vi "doubleshutter_imagesplit.vi"(0 "image array":dbl[][](array[numeric]), 1 "DoubleShutter?":bool, 3 "x bin":dbl) -> (5 "lower half - atoms":dbl[][](graph), 6 "upper half - background":dbl[][](graph), 7 "Uncut Image":dbl[][](graph))   [LabVIEW 2013]
panel:
  in  "y bin":dbl
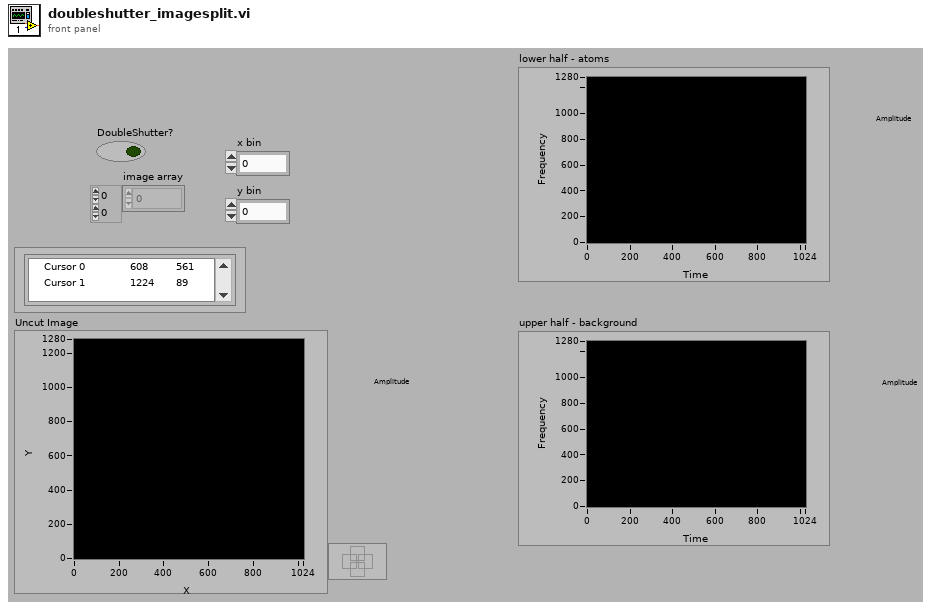
[diagram p1: front panel]
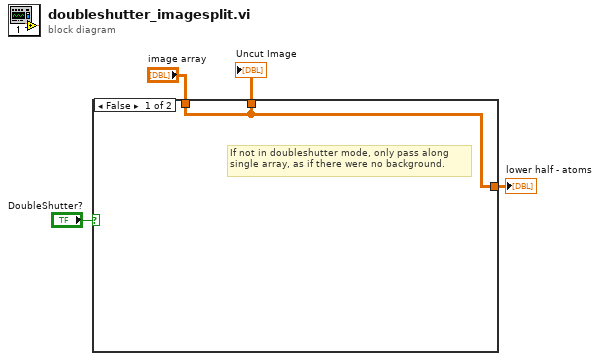
[diagram p0: block diagram]
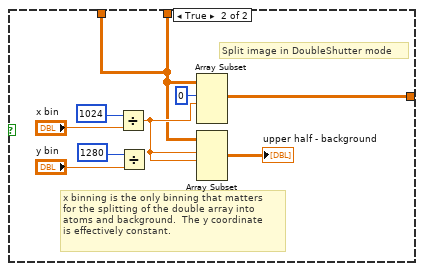
[diagram p2: hidden frame]
diagram:
  n1 = case shown="False" "DoubleShutter?" {
    tunnel: [w5 w8] -> w4
    tunnel: "image array" -> [w5 w8]
    tunnel: [w5 w7] -> w1
    frame False {
      # "If not in doubleshutter mode, only pass along\nsingle array, as if there were no background."
    }
    frame True {
      # "Split image in DoubleShutter mode"
      # "x binning is the only binning that matters\nfor the splitting of the double array into\natoms and background.  The y coordinate\nis effectively constant."
      n2 = Divide(x=1024 ("length"), y="x bin") -> (x/y=w12:dbl)
      n3 = Divide(x=1280 ("length"), y="y bin") -> ()  [unwired: 1 out]
      n4 = Array Subset(array=w8, index (row)=0 ("index"), length (row)=w12) -> (w7:dbl[][])  [unwired: 2 in]
      n5 = Array Subset(array=w8, index (row)=w12, length (row)=w12) -> (→"upper half - background":dbl[][])  [unwired: 2 in]
    }
  }
  "Uncut Image" <- w4
  "lower half - atoms" <- w1
